vi "Set Fully Explored.vi"(8 "Error In":errorcluster, 11 "DFS Data In":T1) -> (0 "Error Out":errorcluster, 3 "DFS Data Out":T1)   [LabVIEW 2022 SP3]
doc: "This VI sets the \"Fully Explored\" flag of the node at the current index."
uses:
  DFS Data (cluster).ctl
  DFS Node (cluster).ctl
  DFS Child Node (cluster).ctl
panel:
  # "Development\nControls or indicators that are useful for development or testing, but which are not outputs of the VI."
  # "Input\nInputs to the VI"
  # "Output\nOutputs of the VI"
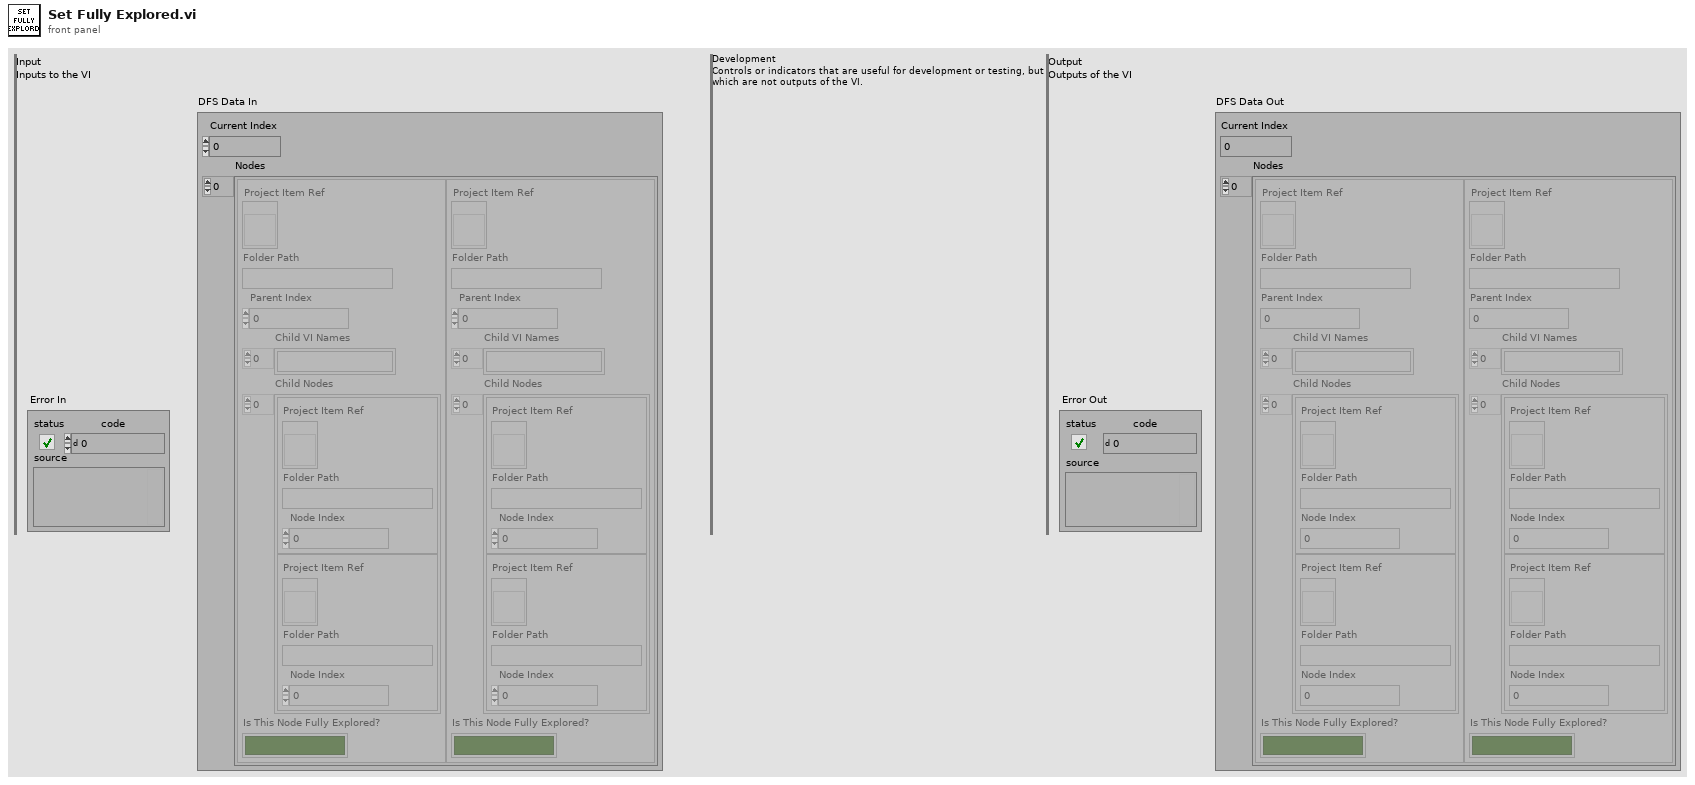
[diagram p1: front panel]
types:
  T1 = typedef "DFS Data (cluster).ctl" = cluster{"Current Index":i32, "Nodes":T2[]}
  T2 = typedef "DFS Node (cluster).ctl" = cluster{"Project Item Ref":refnum<vi>, "Folder Path":string, "Parent Index":i32, "Child VI Names":string[], "Child Nodes":T3[], "Is This Node Fully Explored?":bool}
  T3 = typedef "DFS Child Node (cluster).ctl" = cluster{"Project Item Ref":refnum<vi>, "Folder Path":string, "Node Index":i32}
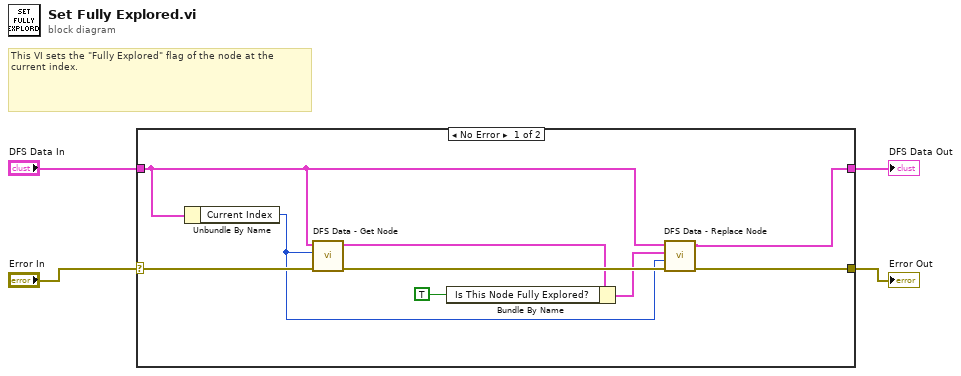
[diagram p0: block diagram]
diagram:
  # "This VI sets the \"Fully Explored\" flag of the node at the current index."
  n1 = case shown="No Error" "Error In" {
    selector: "Error In" -> [w13 w15]
    tunnel: [w11 w15] -> w3
    tunnel: "DFS Data In" -> [w9 w14]
    tunnel: [w10 w14] -> w1
    frame No Error {
      n2 = Unbundle By Name(w9) -> ("Current Index"=w6:i32)
      n3 = call "DFS Data - Get Node.vi"("Error In"=w13, "Node Index"=w6, "DFS Data"=w9) -> ("Error Out"=w12:errorcluster, "DFS Node"=w5:T2)  [unwired: 7 in]
      n4 = Bundle By Name(cluster=w5, "Is This Node Fully Explored?"=TRUE) -> (w7:T2)
      n5 = call "DFS Data - Replace Node.vi"("Error In"=w12, "Node Index"=w6, "New Node Value"=w7, "DFS Data In"=w9) -> ("Error Out"=w11:errorcluster, "DFS Data Out"=w10:T1)  [unwired: 6 in]
    }
    frame Error {
    }
  }
  "Error Out" <- w3
  "DFS Data Out" <- w1
